vi "Calculate Checksum (CRC-16).vi"(0 "Message":string) -> (2 "CRC [String]":string)   [LabVIEW 2023]
doc: "This VI computes the CRC16 CCITT of any message. This implementation was derived from the C code provided by http://www.joegeluso.com/software/articles/ccitt.htm"
panel:
  out "CRC [I32]":i32 format="%x"
  # "POLY 1021"
  # "Initial Value = 0000"
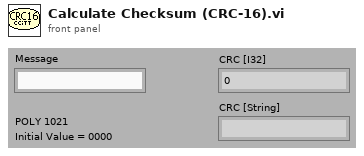
[diagram p1: front panel]
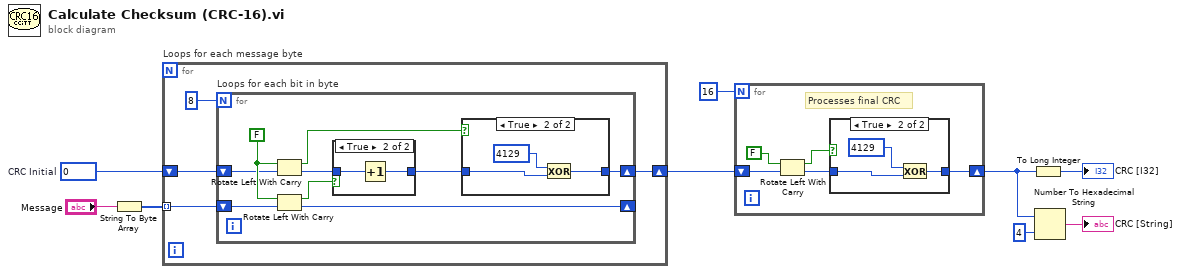
[diagram p0: block diagram]
diagram:
  w8 = u16 0  # CRC Initial
  n1 = String To Byte Array(string="Message") -> (unsigned byte array=w5:u8[])
  n2 = for "Loops for each message byte" {
    tunnel: w5 -> [w12] mode=indexing
    shift-right: [w10] -> w6
    shift-left: w8 -> [w11]
    n3 = for "Loops for each bit in byte" {
      N: 8 -> [_]
      shift-right: [w17] -> _
      shift-left: w12 -> [w16]
      shift-right: [w14] -> w10
      shift-left: w11 -> [w15]
      w18 = FALSE ("carry")
      n4 = Rotate Left With Carry(2:w15, 3:w18) -> (0:w21:u16, 1:w22:bool)
      n5 = Rotate Left With Carry(2:w16, 3:w18) -> (0:w17:u8, 1:w19:bool)
      n6 = case shown="True" w19 {
        tunnel: [w23 w24] -> w20
        tunnel: w21 -> [w23 w25]
        frame False {
        }
        frame True {
          n7 = Increment(x=w25) -> (x+1=w24:u16)
        }
      }
      n8 = case shown="True" w22 {
        tunnel: w20 -> [w26 w28]
        tunnel: [w26 w27] -> w14
        frame False {
        }
        frame True {
          n9 = Exclusive Or(1:w28, 2:u16 4129) -> (0:w27:u16)
        }
      }
    }
  }
  n10 = for {
    N: 16 -> [_]
    shift-right: [w32] -> w3
    shift-left: w6 -> [w31]
    # "Processes final CRC"
    n11 = Rotate Left With Carry(2:w31, 3:FALSE ("carry")) -> (0:w30:u16, 1:w34:bool)
    n12 = case shown="True" w34 {
      tunnel: w30 -> [w35 w36]
      tunnel: [w35 w37] -> w32
      frame False {
      }
      frame True {
        n13 = Exclusive Or(1:w36, 2:u16 4129) -> (0:w37:u16)
      }
    }
  }
  n14 = To Long Integer(number=w3) -> (32bit integer=→"CRC [I32]":i32)
  n15 = Number To Hexadecimal String(1:i16 4 ("width (-)"), 2:w3) -> (0:→"CRC [String]":string)
